vi "Get Module Names.vi"() -> (3 "Module Names":string[](array[string]))   [LabVIEW 2017, in "Scan Engine Custom Device.lvlib"]
uses:
  Scan Engine Custom Device.lvlib
  Modules.lvlibp/RSI Module/Module Models.ctl
  Modules.lvlibp/RSI Module/RSI Module.lvclass
panel:
  in  "Module Typedef":T1
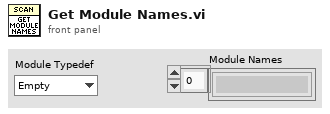
[diagram p1: front panel]
types:
  T1 = typedef "Modules.lvlibp/RSI Module.lvclass/Module Models.ctl" = enum16{"Empty", "NI 9201", "NI 9203", "NI 9205", "NI 9206", "NI 9207", "NI 9208", "NI 9211", "NI 9212", "NI 9213", "NI 9214", "NI 9215", "NI 9217", "NI 9219", "NI 9220", "NI 9221", "NI 9222", "NI 9223", "NI 9225", "NI 9227", "NI 9229", "NI 9233", "NI 9234", "NI 9235", "NI 9236", "NI 9237", "NI 9239", "NI 9242", "NI 9244", "NI 9263", "NI 9264", "NI 9265", "NI 9269", "NI 9375", "NI 9401", "NI 9402", "NI 9403", "NI 9411", "NI 9421", "NI 9422", "NI 9423", "NI 9425", "NI 9426", "NI 9435", "NI 9437", "NI 9472", "NI 9474", "NI 9475", "NI 9476", "NI 9477", "NI 9478", "NI 9481", "NI 9482", "NI 9485", "NI 9266"}
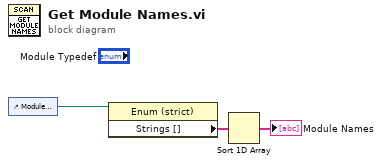
[diagram p0: block diagram]
diagram:
  n1 = control-ref of="Module Typedef"() -> (w2:refnum<vi>)
  n2 = property class="Enum (strict)"(reference=w2) -> ("Strings []"=w3:string[])  [unwired: 1 in, 2 out]
  n3 = Sort 1D Array(array=w3) -> (sorted array=→"Module Names":string[])
